vi "Set Debug Flags.vi"(10 "Debug Flags":refnum<class "Debug Flags.lvclass">, 11 "Transceiver Thread in":refnum<class "Transceiver Thread.lvclass">) -> (3 "Transceiver Thread out":refnum<class "Transceiver Thread.lvclass">)   [LabVIEW 2017, in "Data Sharing Framework Engine.lvlib" / "Transceiver Thread.lvclass"]
uses:
  Transceiver Thread.lvclass
  Debug/Debug Flags/Debug Flags.lvclass
  Transceiver Thread.lvclass/Transceiver Thread.ctl
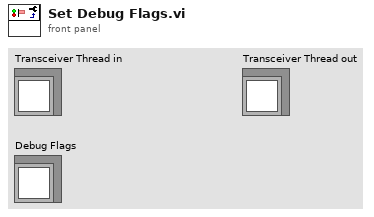
[diagram p1: front panel]
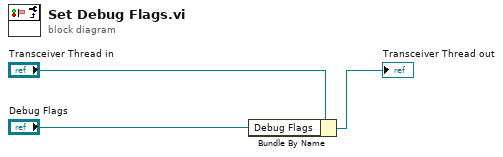
[diagram p0: block diagram]
diagram:
  n1 = Bundle By Name(cluster="Transceiver Thread in", "Debug Flags"="Debug Flags") -> (→"Transceiver Thread out":refnum<class "Transceiver Thread.lvclass">)
